vi "Core Action.vi"(8 "error in (no error)":errorcluster, 10 "SECS-II Class":refnum<class "SECS-II Class.lvclass">, 11 "14-Process Program Creating Editing or Deleting in":refnum<class "14-Process Program Creating Editing or Deleting.lvclass">) -> (0 "error out":errorcluster, 2 "SECS-II Class Out":refnum<class "SECS-II Class.lvclass">, 3 "14-Process Program Creating Editing or Deleting out":refnum<class "14-Process Program Creating Editing or Deleting.lvclass">)   [LabVIEW 2020, in "SECS Scenarios.lvlib" / "14-Process Program Creating Editing or Deleting.lvclass"]
uses:
  14-Process Program Creating Editing or Deleting.lvclass
  D:/Dropbox/SECS/SECS_GEM v1.1.0/Com/SECS Scenarios/Scenarios Class/Scenarios Class.lvclass
  SECS Communication/SECS-II Class/SECS-II Class.lvclass
  14-Process Program Creating Editing or Deleting.lvclass/14-Process Program Creating Editing or Deleting.ctl
  Scenarios Class/Scenarios Class.lvclass
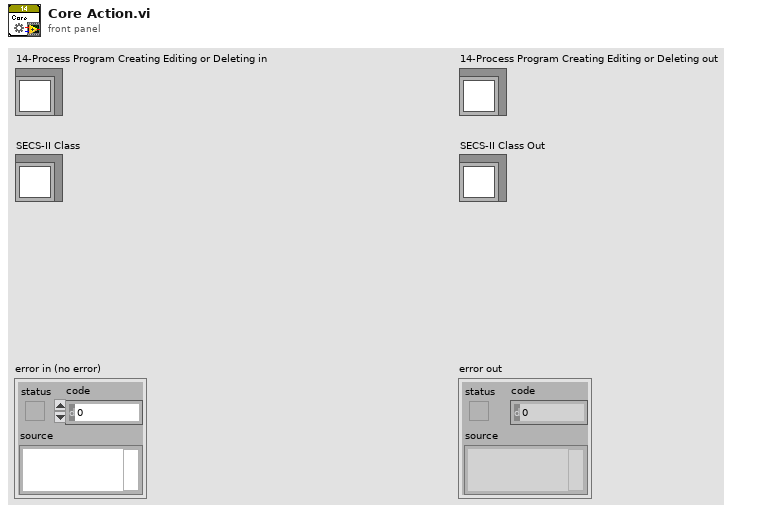
[diagram p1: front panel]
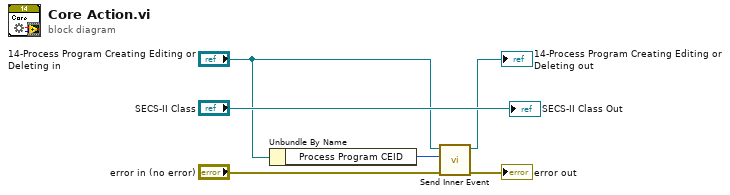
[diagram p0: block diagram]
diagram:
  n1 = Unbundle By Name("14-Process Program Creating Editing or Deleting in") -> ("Process Program CEID"=w4:u32)
  n2 = call "Send Inner Event.vi"("error in (no error)"="error in (no error)", "CEID"=w4, "Scenarios Class in"="14-Process Program Creating Editing or Deleting in") -> ("error out"=→"error out":errorcluster, "Scenarios Class out"=→"14-Process Program Creating Editing or Deleting out":refnum<class "14-Process Program Creating Editing or Deleting.lvclass">)  [unwired: 7 in]
  "SECS-II Class Out" <- "SECS-II Class"
